vi "Task9.vi"() -> ()   [LabVIEW 2017]
panel:
  out "Array":string[](array[string])
  in  "String":string
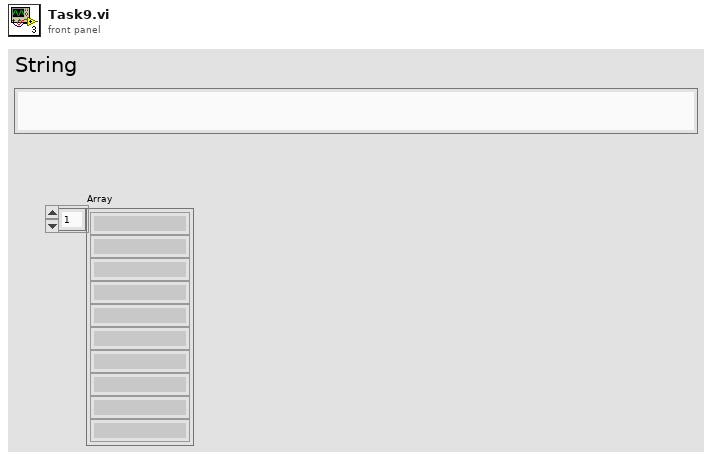
[diagram p1: front panel]
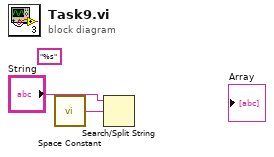
[diagram p0: block diagram]
diagram:
  (unwired) "%s"
  n1 = call <vilib>:"Space Constant.vi"() -> ("String"=w2:string)
  n2 = Search/Split String(string="String", search string/char (-)=w2) -> ()  [unwired: 1 in, 3 out]
